vi "recondense_Merge_Cluster.vi"(1 "Recondense-Control":T1, 2 "Recondense-Status":T2) -> (0 "Recondense-Monitor":T3 {"He3-Pot Heater %" format="%#_4g"; "He3-Pot Setpoint" format="%#_4g"; "Sorb Heater %" format="%#_4g"; "Sorb Setpoint" format="%#_4g"; "He3 Temp2" format="%#_4g"; "He3 Temp 1" format="%#_4g"; "1K Temp" format="%#_4g"; "Sorb Temp" format="%#_4g"})   [LabVIEW 2019]
uses:
  Brosowski/BorowskiMonitor.ctl
  Brosowski/Borowski-Status-Cluster.ctl
  Brosowski/Borowski-Control-Cluster.ctl
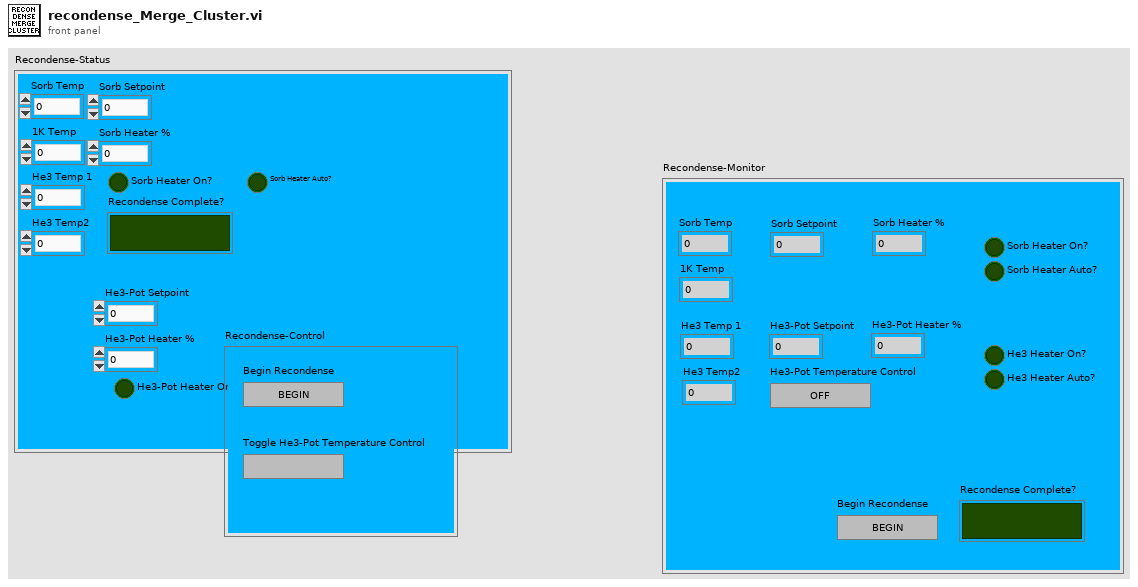
[diagram p1: front panel]
types:
  T1 = typedef "Borowski-Control-Cluster.ctl" = cluster{"Begin Recondense":bool, "Toggle He3-Pot Temperature Control":bool}
  T2 = typedef "Borowski-Status-Cluster.ctl" = cluster{"Sorb Temp":dbl, "1K Temp":dbl, "He3 Temp 1":dbl, "He3 Temp2":dbl, "Recondense Complete?":bool, "Sorb Heater Auto?":bool, "Sorb Heater On?":bool, "Sorb Setpoint":dbl, "Sorb Heater %":dbl, "He3-Pot Heater Auto?":bool, "He3-Pot Heater On?":bool, "He3-Pot Setpoint":dbl, "He3-Pot Heater %":dbl}
  T3 = typedef "BorowskiMonitor.ctl" = cluster{"Sorb Temp":dbl, "1K Temp":dbl, "He3 Temp 1":dbl, "He3 Temp2":dbl, "Recondense Complete?":bool, "Sorb Heater Auto?":bool, "Sorb Heater On?":bool, "Sorb Setpoint":dbl, "Sorb Heater %":dbl, "Begin Recondense":bool, "He3-Pot Setpoint":dbl, "He3-Pot Heater %":dbl, "He3 Heater Auto?":bool, "He3 Heater On?":bool, "He3-Pot Temperature Control":bool}
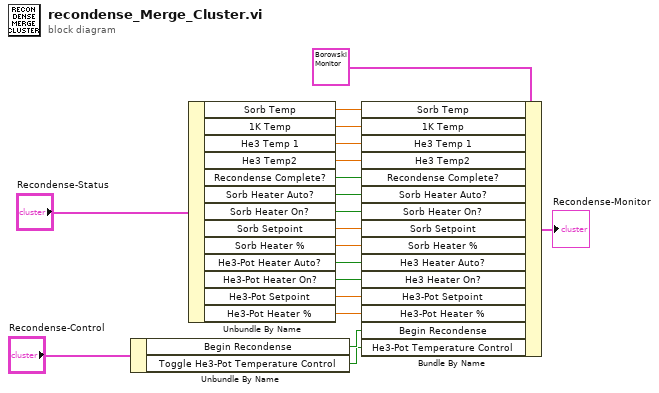
[diagram p0: block diagram]
diagram:
  n1 = Unbundle By Name("Recondense-Control") -> ("Begin Recondense"=w6:bool, "Toggle He3-Pot Temperature Control"=w5:bool)
  n2 = Unbundle By Name("Recondense-Status") -> ("Sorb Temp"=w16:dbl, "1K Temp"=w15:dbl, "He3 Temp 1"=w14:dbl, "He3 Temp2"=w13:dbl, "Recondense Complete?"=w12:bool, "Sorb Heater Auto?"=w11:bool, "Sorb Heater On?"=w10:bool, "Sorb Setpoint"=w9:dbl, "Sorb Heater %"=w8:dbl, "He3-Pot Heater Auto?"=w4:bool, "He3-Pot Heater On?"=w3:bool, "He3-Pot Setpoint"=w2:dbl, "He3-Pot Heater %"=w1:dbl)
  n3 = Bundle By Name(cluster=T3 {"Sorb Temp"=0.0, "1K Temp"=0.0, "He3 Temp 1"=0.0, "He3 Temp2"=0.0, "Recondense Complete?"=FALSE, "Sorb Heater Auto?"=FALSE, "Sorb Heater On?"=FALSE, "Sorb Setpoint"=0.0, "Sorb Heater %"=0.0, "Begin Recondense"=FALSE, "He3-Pot Setpoint"=0.0, "He3-Pot Heater %"=0.0, "He3 Heater Auto?"=FALSE, "He3 Heater On?"=FALSE, "He3-Pot Temperature Control"=FALSE} ("Recondense-Monitor"), "Sorb Temp"=w16, "1K Temp"=w15, "He3 Temp 1"=w14, "He3 Temp2"=w13, "Recondense Complete?"=w12, "Sorb Heater Auto?"=w11, "Sorb Heater On?"=w10, "Sorb Setpoint"=w9, "Sorb Heater %"=w8, "He3 Heater Auto?"=w4, "He3 Heater On?"=w3, "He3-Pot Setpoint"=w2, "He3-Pot Heater %"=w1, "Begin Recondense"=w6, "He3-Pot Temperature Control"=w5) -> (→"Recondense-Monitor":T3)
